vi "OAT Compensate Vector Data.vi"   [LabVIEW 2017, in "SoundVib_RefDataProcess.lvlib"]
doc: "Compensates for the shaft bow and electrical variations in displacement transducer signals. This VI performs slow-roll compensation by subtracting <B>vector references</B> from the corresponding <B>magnitudes [RMS]</B> and <B>phases [phase lag]</B>. Wire data to the <B>magnitudes [RMS]</B> and <B>phases [phase lag]</B> inputs to determine the polymorphic instance to use or manually select the instance."
uses:
  <vilib>/addons/Sound and Vibration/Order Analysis/Referece Data Processing/SoundVib_RefDataProcess.lvlib
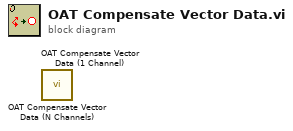
[diagram p0: block diagram]
diagram:
  n1 = call <vilib>:"OAT Compensate Vector Data (N Channels).vi"() -> ()  [unwired: 12 in, 4 out]
  n2 = call <vilib>:"OAT Compensate Vector Data (1 Channel).vi"() -> ()  [unwired: 12 in, 4 out]
